vi "Initialize Starting Tab.vi"(8 "error in (no error)":errorcluster, 11 "Numeric Data Type in":refnum<class "Numeric Data Type.lvclass">) -> (0 "error out":errorcluster, 3 "Numeric Data Type out":refnum<class "Numeric Data Type.lvclass">)   [LabVIEW 2018, in "Numeric Data Type.lvclass"]
uses:
  Numeric Data Type.lvclass
  Reference Main Tab.vi
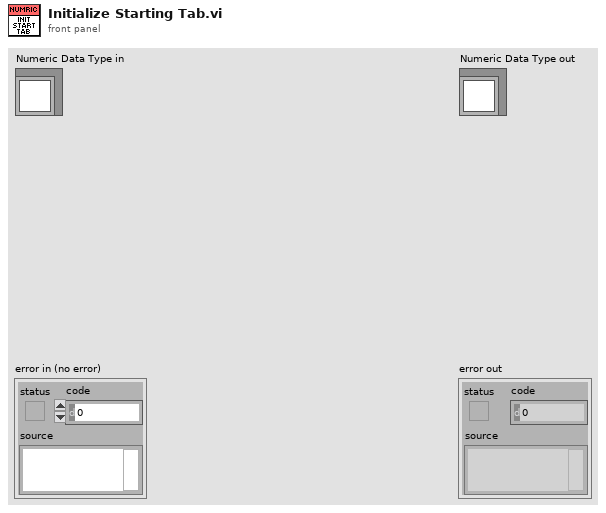
[diagram p1: front panel]
types:
  T1 = enum32{"Column Format", "Data Type", "Data Entry", "Display Format"}
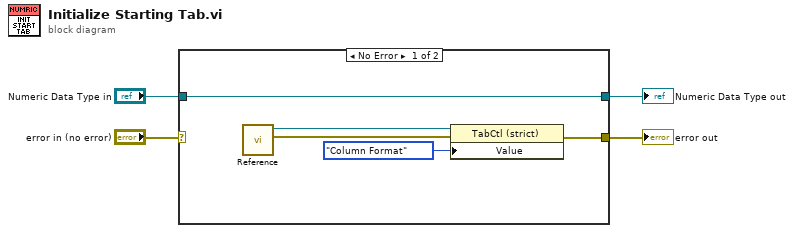
[diagram p0: block diagram]
diagram:
  n1 = case shown="No Error" "error in (no error)" {
    selector: "error in (no error)" -> [_ w11]
    tunnel: [w7 w11] -> w3
    tunnel: [w9 w10] -> w1
    tunnel: "Numeric Data Type in" -> [w9 w10]
    frame No Error {
      n2 = call-poly "Reference.vi"() -> ("error out"=w6:errorcluster, "Main Tab"=w8:refnum<vi>)  [unwired: 10 in]
      n3 = property class="TabCtl (strict)"(reference=w8, error in=w6, "Value"=T1."Column Format") -> (error out=w7:errorcluster)  [unwired: 1 out]
    }
    frame Error {
    }
  }
  "error out" <- w3
  "Numeric Data Type out" <- w1
